vi "MB Ethernet Connection Manager.vi"(7 "Function":T1, 10 "Priority":bool, 11 "Connection ID":refnum<k5>) -> (1 "Close Connection":bool, 2 "Connection IDs":refnum<k5>[](array[refnum]), 3 "Connection ID to Delete":refnum<k5>)   [LabVIEW 2023, in "Voegtlin_NI_SMART_Modbus_Drivers.lvlib"]
uses:
  Voegtlin_NI_SMART_Modbus_Drivers.lvlib
  MB Ethernet Connection Function.ctl
  MB Globals.vi
panel:
  # "VI Name: MB Ethernet Connection Manager.vi\nPurpose: Connection ID manager.\nThis VI manages Connection IDs (add, get, delete, etc..)\nThis is a critical resource, so the VI is set to Subroutine to prevent from being accessed by several VIs at a time."
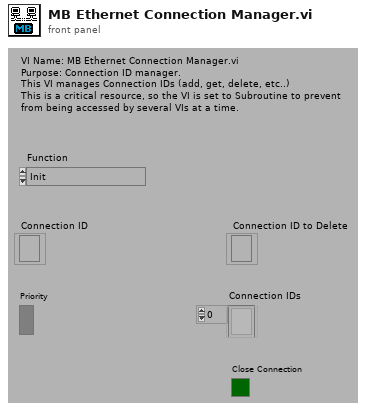
[diagram p1: front panel]
types:
  T1 = typedef "Voegtlin_NI_SMART_Modbus_Drivers.lvlib/MB Ethernet Connection Function.ctl" = enum16{"Init", "Add Connection", "Get All Connections", "Delete Connection"}
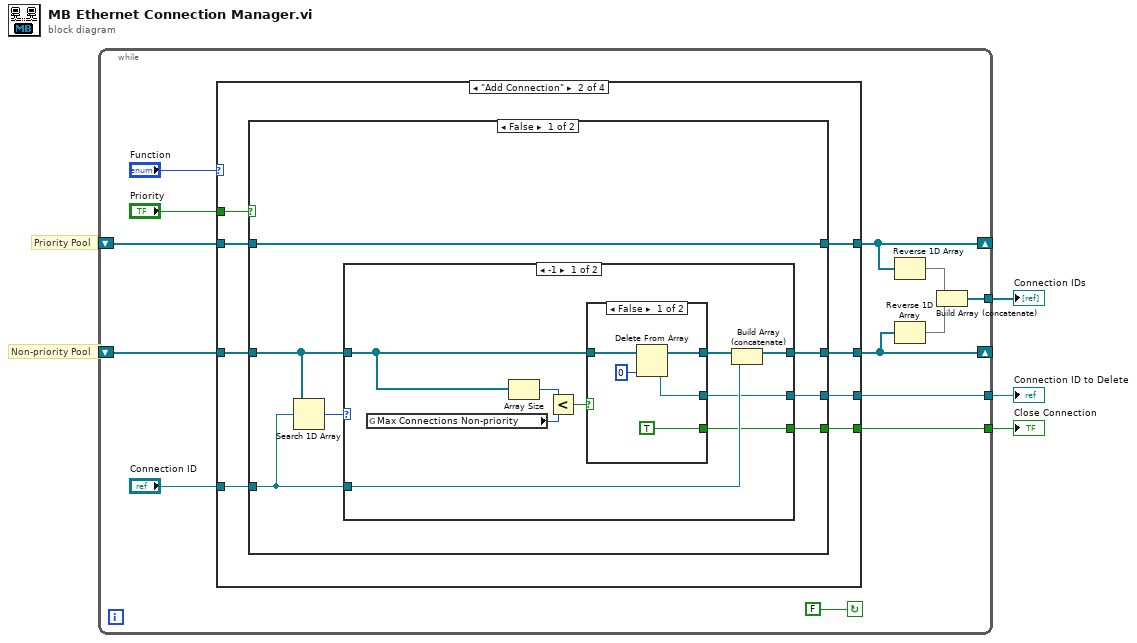
[diagram p0: block diagram]
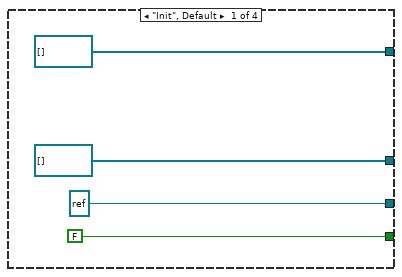
[diagram p2: hidden frame]
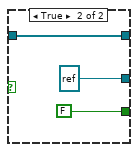
[diagram p3: hidden frame]
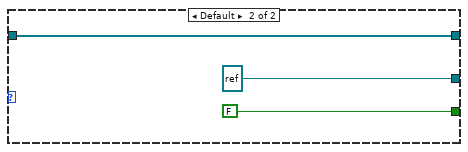
[diagram p4: hidden frame]
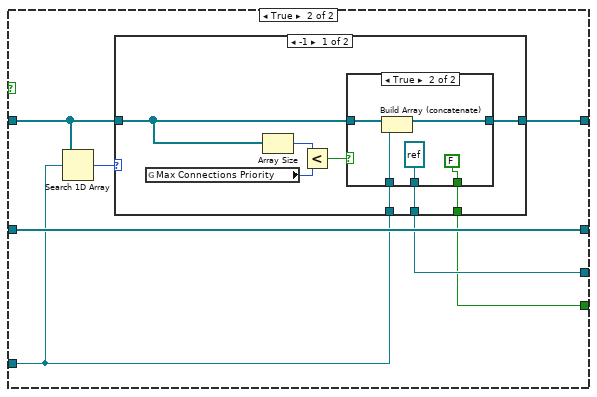
[diagram p5: hidden frame]
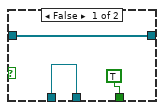
[diagram p6: hidden frame]
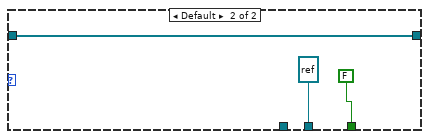
[diagram p7: hidden frame]
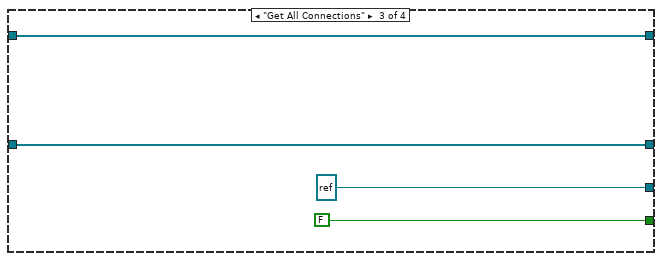
[diagram p8: hidden frame]
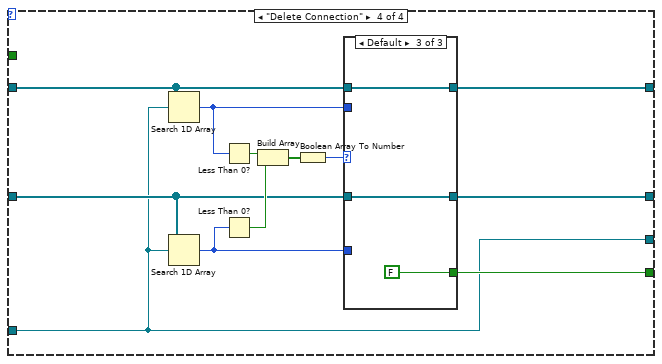
[diagram p9: hidden frame]
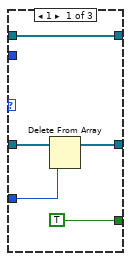
[diagram p10: hidden frame]
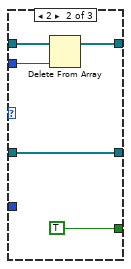
[diagram p11: hidden frame]
diagram:
  # "Non-priority Pool"
  # "Priority Pool"
  n1 = while {
    shift-right: [w5] -> _
    shift-left: _ -> [w15]
    shift-right: [w7] -> _
    shift-left: _ -> [w14]
    tunnel: [w11] -> w1
    tunnel: [w9] -> w3
    tunnel: [w8] -> w2
    stop <- FALSE continue-if-true
    n2 = case shown="\"Add Connection\"" "Function" {
      tunnel: [refnum<k5>[] [] w26 w85 w90] -> w5
      tunnel: [refnum<k5>[] [] w27 w84 w92] -> w7
      tunnel: w15 -> [_ w24 w85 w91]
      tunnel: w14 -> [_ w23 w84 w93]
      tunnel: "Priority" -> [_ w28 _ _]
      tunnel: "Connection ID" -> [_ w25 _ w86]
      tunnel: [refnum<k5> refnum ("TCP Connection Refnum") w22 refnum<k5> refnum ("TCP Connection Refnum") w86] -> w9
      tunnel: [FALSE w21 FALSE w87] -> w8
      frame "Init", Default {
      }
      frame "Add Connection" {
        n3 = case shown="False" w28 {
          tunnel: w24 -> [w34 w60]
          tunnel: w23 -> [w30 w61]
          tunnel: w25 -> [w29 w59]
          tunnel: [w35 w61] -> w27
          tunnel: [w34 w62] -> w26
          tunnel: [w33 w57] -> w22
          tunnel: [w32 w56] -> w21
          frame False {
            n4 = Search 1D Array(1D array=w30, element=w29) -> (index of element=w31:i32)  [unwired: 1 out]
            n5 = case shown="-1" w31 {
              tunnel: [w44 w55] -> w35
              tunnel: w30 -> [w40 w55]
              tunnel: w29 -> [w38 _]
              tunnel: [w37 refnum<k5> refnum ("TCP Connection Refnum")] -> w33
              tunnel: [w36 FALSE] -> w32
              frame -1 {
                n6 = global read "MB Globals.vi" "Max Connections Non-priority"() -> (w42:i32)
                n7 = Array Size(array=w40) -> (size(s)=w43:i32)
                n8 = Less?(x=w43, y=w42) -> (x < y?=w41:bool)
                n9 = case shown="False" w41 {
                  tunnel: w40 -> [w49 w52]
                  tunnel: [w48 w52] -> w39
                  tunnel: [w46 refnum<k5> refnum ("TCP Connection Refnum")] -> w37
                  tunnel: [TRUE FALSE] -> w36
                  frame False {
                    n10 = Delete From Array(array=w49, index=0) -> (deleted portion=w46:refnum<k5>, array with subset deleted=w48:refnum<k5>[])  [unwired: 1 in]
                  }
                  frame True {
                  }
                }
                n11 = Build Array (concatenate)(w39, w38) -> (w44:refnum<k5>[])
              }
              frame Default {
              }
            }
          }
          frame True {
            n12 = Search 1D Array(1D array=w60, element=w59) -> (index of element=w58:i32)  [unwired: 1 out]
            n13 = case shown="-1" w58 {
              tunnel: [w68 w81] -> w62
              tunnel: w60 -> [w66 w81]
              tunnel: w59 -> [w65 _]
              tunnel: [w64 refnum<k5> refnum ("TCP Connection Refnum")] -> w57
              tunnel: [w63 FALSE] -> w56
              frame -1 {
                n14 = global read "MB Globals.vi" "Max Connections Priority"() -> (w69:i32)
                n15 = Array Size(array=w66) -> (size(s)=w70:i32)
                n16 = Less?(x=w70, y=w69) -> (x < y?=w67:bool)
                n17 = case shown="True" w67 {
                  tunnel: w65 -> [w72 w78]
                  tunnel: [w73 w77] -> w68
                  tunnel: w66 -> [w73 w76]
                  tunnel: [w72 refnum<k5> refnum ("TCP Connection Refnum")] -> w64
                  tunnel: [TRUE FALSE] -> w63
                  frame False {
                  }
                  frame True {
                    n18 = Build Array (concatenate)(w76, w78) -> (w77:refnum<k5>[])
                  }
                }
              }
              frame Default {
              }
            }
          }
        }
      }
      frame "Get All Connections" {
      }
      frame "Delete Connection" {
        n19 = Search 1D Array(1D array=w91, element=w86) -> (index of element=w89:i32)  [unwired: 1 out]
        n20 = Search 1D Array(1D array=w93, element=w86) -> (index of element=w88:i32)  [unwired: 1 out]
        n21 = Less Than 0?(x=w89) -> (x < 0?=w97:bool)
        n22 = Less Than 0?(x=w88) -> (x < 0?=w96:bool)
        n23 = Build Array(w97, w96) -> (w95:bool[])
        n24 = Boolean Array To Number(Boolean array=w95) -> (number=w94:u32)
        n25 = case shown="Default" w94 {
          tunnel: w93 -> [w102 w104 w109]
          tunnel: [w101 w104 w109] -> w92
          tunnel: w91 -> [w99 w107 w110]
          tunnel: [w99 w105 w110] -> w90
          tunnel: w89 -> [_ w106 _]
          tunnel: w88 -> [w100 _ _]
          tunnel: [TRUE TRUE FALSE] -> w87
          frame 1 {
            n26 = Delete From Array(array=w102, index=w100) -> (array with subset deleted=w101:refnum<k5>[])  [unwired: 1 in, 1 out]
          }
          frame 2 {
            n27 = Delete From Array(array=w107, index=w106) -> (array with subset deleted=w105:refnum<k5>[])  [unwired: 1 in, 1 out]
          }
          frame Default {
          }
        }
      }
    }
    n28 = Reverse 1D Array(array=w5) -> (reversed array=w6:refnum<k5>[])
    n29 = Reverse 1D Array(array=w7) -> (reversed array=w4:refnum<k5>[])
    n30 = Build Array (concatenate)(w6, w4) -> (w11:refnum<k5>[])
  }
  "Connection IDs" <- w1
  "Connection ID to Delete" <- w3
  "Close Connection" <- w2
